vi "ATI-UDP-Client.vi"() -> ()   [LabVIEW 2021]
uses:
  <vilib>/Utility/file.llb/Write To Spreadsheet File (DBL).vi
panel:
  in  "Save Input Data to File":bool=TRUE
  in  "Data File":path
  out "Measurement":dbl[][](graph) caption="F/T Data"
  out "F/T":dbl[][](array[numeric]) format="%0.2f"
  in  "Stop":bool
  # "Stop Receiving UDP Data"
  # "ON"
  # "OFF"
  # "Resolved Force/Torque Readings from Server.  These are the first few \nrecords from the most recent set.  To see more records,\nexpand this array vertically, or set the major index."
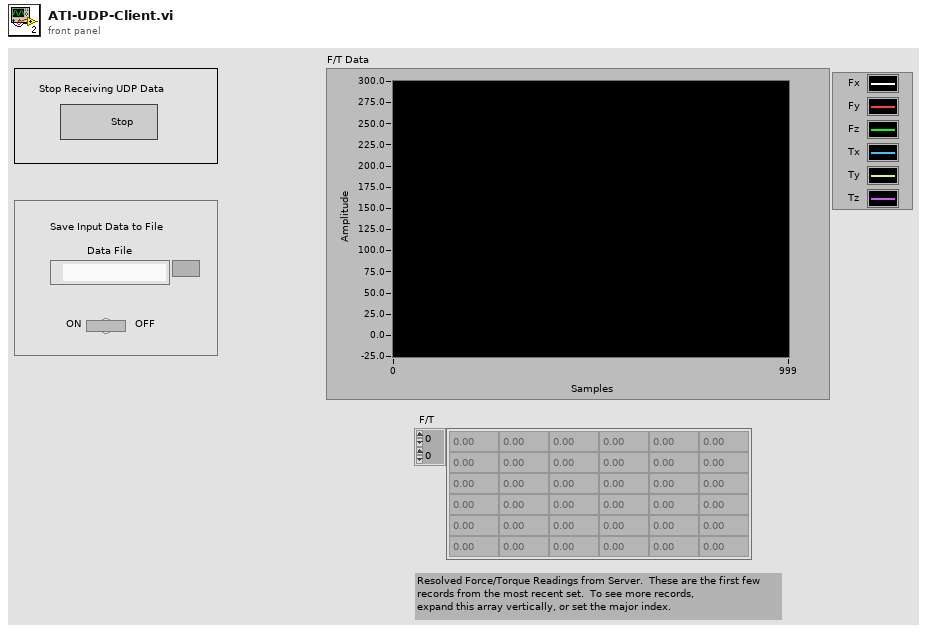
[diagram p1: front panel]
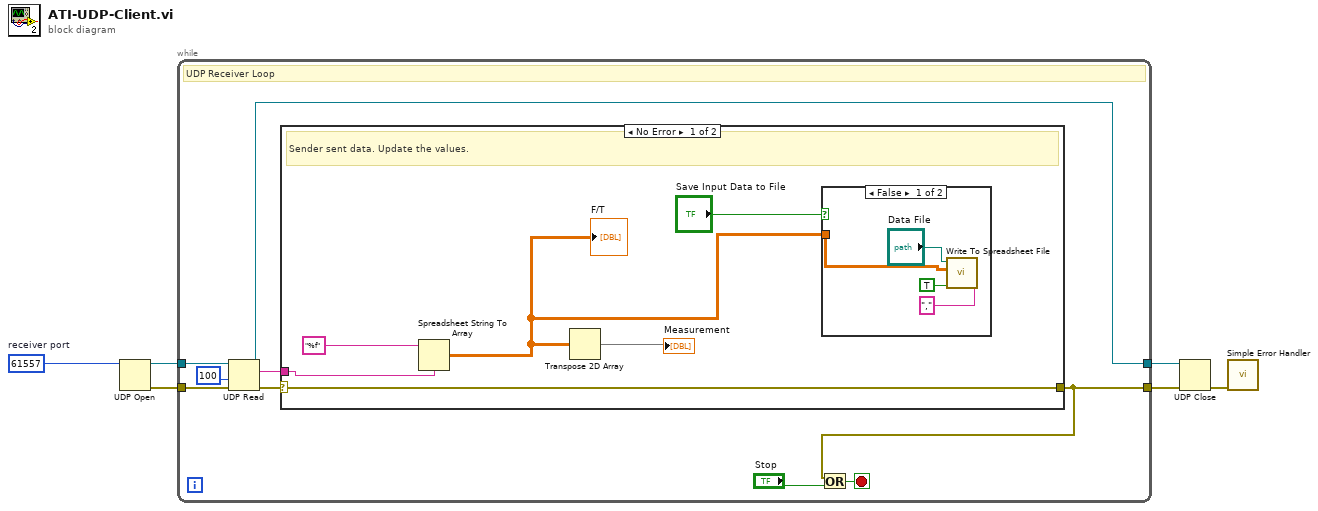
[diagram p0: block diagram]
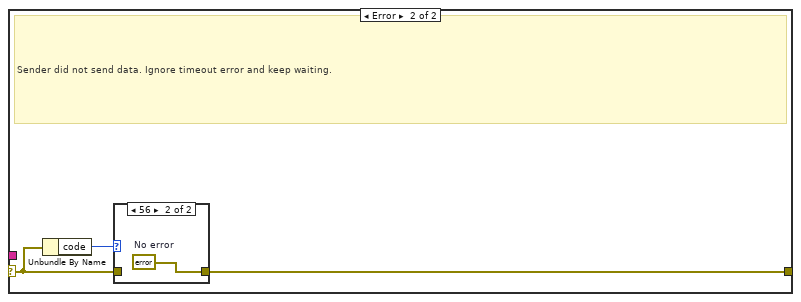
[diagram p3: hidden frame]
diagram:
  w1 = u16 61557  # receiver port
  n1 = UDP Open(11:w1) -> (port=w2:refnum<k16>, 0:w3:errorcluster)  [unwired: 4 in, 1 out]
  n2 = while {
    tunnel: w2 -> [w15]
    tunnel: [w7] -> w6
    tunnel: w3 -> [w12]
    tunnel: [w8] -> w4
    stop <- w13 stop-if-true
    # "UDP Receiver Loop"
    n3 = UDP Read(connection ID=w15, timeout ms (25000)=100, 8:w12) -> (data out=w10:string, error out=w9:errorcluster, 3:w7:refnum<k16>)  [unwired: 3 out]
    n4 = case shown="No Error" w9 {
      selector: w9 -> [w21 w27]
      tunnel: w10 -> [w16 _]
      tunnel: [w21 w26] -> w8
      frame No Error {
        # "Sender sent data. Update the values."
        n5 = Spreadsheet String To Array(delimiter (Tab)=w16, format string="%f") -> (array=w17:dbl[][])  [unwired: 2 in]
        "F/T" <- w17
        n6 = Transpose 2D Array(2D array=w17) -> (transposed array=→"Measurement":dbl[][])
        n7 = case shown="False" "Save Input Data to File" {
          tunnel: w17 -> [w22 _]
          frame False {
            n8 = call-poly <vilib>:"Write To Spreadsheet File.vi"("delimiter (\\t)"=",", "append to file? (new file:F)"=TRUE, "2D data"=w22, "file path (dialog if empty)"="Data File") -> ()  [unwired: 4 in, 1 out]
          }
          frame True {
          }
        }
      }
      frame Error {
        # "Sender did not send data. Ignore timeout error and keep waiting."
        n9 = Unbundle By Name(w27) -> ("code"=w28:i32)
        n10 = case shown="56" w28 {
          tunnel: w27 -> [w29 _]
          tunnel: [w29 w30] -> w26
          frame Default {
          }
          frame 56 {
            w30 = errorcluster {"status"=FALSE, "code"=0, "source"=""}  # No error
          }
        }
      }
    }
    n11 = Or(x=w8, y="Stop") -> (x .or. y?=w13:bool)
  }
  n12 = UDP Close(connection ID=w6, 8:w4) -> (error out=w5:errorcluster)  [unwired: 1 out]
  n13 = call <vilib>:"Simple Error Handler.vi"("error in (no error)"=w5) -> ()  [unwired: 1 in, 8 out]
